vi "Half Adder.vi"(2 "b":bool, 3 "a":bool) -> (0 "c":bool, 1 "s":bool)   [LabVIEW 2012]
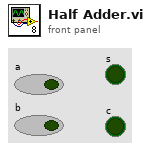
[diagram p1: front panel]
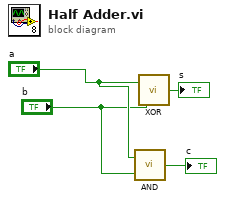
[diagram p0: block diagram]
diagram:
  n1 = call "AND.vi"("b"="b", "a"="a") -> ("x"=→"c":bool)
  n2 = call "XOR.vi"("b"="b", "a"="a") -> ("x"=→"s":bool)
